vi "Close vi references.vi"(8 "error in":errorcluster, 11 "Data Cluster":T1) -> (0 "error out":errorcluster)   [LabVIEW 2019, in "Panther Dashboard.lvlib"]
uses:
  Panther Dashboard.lvlib
  Class/Library/Library.lvclass
  Class/Project/Project.lvclass
  Module type--enum.ctl
  Module Data--cluster.ctl
  <vilib>/National Instruments/Tree Map/Tree Map Data.ctl
  <vilib>/National Instruments/Tree Map/Tree Map.lvlib
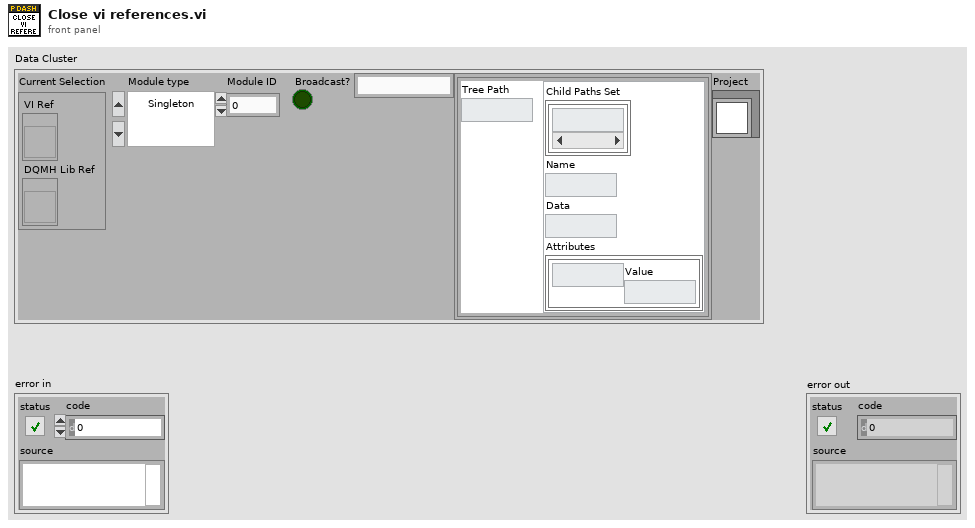
[diagram p1: front panel]
types:
  T1 = typedef "Panther Dashboard.lvlib/Module Data--cluster.ctl" = cluster{"Current Selection":cluster{"VI Ref":refnum<vi>, "DQMH Lib Ref":refnum<vi>}, "Module type":T2, "Module ID":i32, "Broadcast?":bool, "Tree Selection":string, "Tree Map":T3, "Project":refnum<class "Project.lvclass">}
  T2 = typedef "Panther Dashboard.lvlib/Module type--enum.ctl" = enum16{"Singleton", "Cloneable"}
  T3 = typedef "Tree Map.lvlib/Tree Map Data.ctl" = map{string, cluster{"Child Paths Set":set{string}, "Name":string, "Data":string, "Attributes":map{string, string}}}
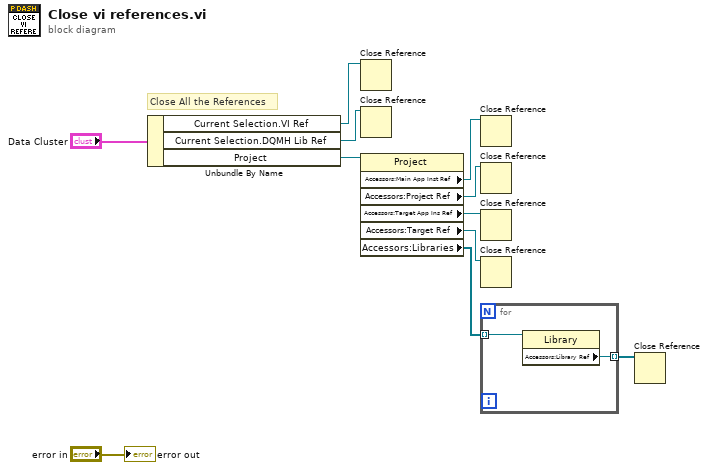
[diagram p0: block diagram]
diagram:
  # "Close All the References"
  n1 = Unbundle By Name("Data Cluster") -> ("Current Selection.VI Ref"=w9:refnum<vi>, "Current Selection.DQMH Lib Ref"=w8:refnum<vi>, "Project"=w7:refnum<class "Project.lvclass">)
  n2 = Close Reference(reference=w9) -> ()  [unwired: 1 in, 1 out]
  n3 = Close Reference(reference=w8) -> ()  [unwired: 1 in, 1 out]
  n4 = property class="Project"(reference=w7) -> ("Accessors:Main App Inst Ref"=w4:refnum<vi>, "Accessors:Project Ref"=w3:refnum<vi>, "Accessors:Target App Ins Ref"=w2:refnum<vi>, "Accessors:Target Ref"=w1:refnum<vi>, "Accessors:Libraries"=w6:refnum<class "Library.lvclass">[])  [unwired: 1 in, 2 out]
  n5 = Close Reference(reference=w4) -> ()  [unwired: 1 in, 1 out]
  n6 = Close Reference(reference=w3) -> ()  [unwired: 1 in, 1 out]
  n7 = Close Reference(reference=w2) -> ()  [unwired: 1 in, 1 out]
  n8 = Close Reference(reference=w1) -> ()  [unwired: 1 in, 1 out]
  n9 = for {
    tunnel: w6 -> [w13] mode=indexing
    tunnel: [w12] -> w5 mode=indexing
    n10 = property class="Library"(reference=w13) -> ("Accessors:Library Ref"=w12:refnum<vi>)  [unwired: 1 in, 2 out]
  }
  n11 = Close Reference(reference=w5) -> ()  [unwired: 1 in, 1 out]
  "error out" <- "error in"
